vi "U3 eGetS Example.vi"() -> (0 "error out":errorcluster)   [LabVIEW 2020]
panel:
  in  "IOType":string="LJ_ioGET_AIN"
  in  "x1":i32=32
  in  "FirstFound":bool=TRUE
  in  "Address":string="1"
  in  "Value Write":dbl format="%.3f"
  out "Error Message":string="No Error"
  out "Value Read":dbl format="%.6f"
  in  "Channel #":i32
  # "IOTypes:\n\nLJ_ioGET_AIN = 10\nLJ_ioGET_AIN_DIFF = 15\nLJ_ioGET_AIN_ADVANCED = 16\nLJ_ioPUT_AIN_RANGE = 2000\nLJ_ioGET_AIN_RANGE = 2001\nLJ_ioPUT_ANALOG_ENABLE_BIT = 2013\nLJ_ioGET_ANALOG_ENABLE_BIT = 2014\nLJ_ioPUT_ANALOG_ENABLE_PORT = 2015\nLJ_ioGET_ANALOG_ENABLE_PORT = 2016\nLJ_ioPUT_DAC = 20\nLJ_ioPUT_DAC_ENABLE = 2002\nLJ_ioGET_DAC_ENABLE = 2003\nLJ_ioGET_DIGITAL_BIT = 30\nLJ_ioGET_DIGITAL_BIT_DIR = 31\nLJ_ioGET_DIGITAL_BIT_STATE = 32\nLJ_ioGET_DIGITAL_PORT = 35\nLJ_ioGET_DIGITAL_PORT_DIR = 36\nLJ_ioGET_DIGITAL_PORT_STATE = 37\nLJ_ioPUT_DIGITAL_BIT = 40\nLJ_ioPUT_DIGITAL_PORT = 45\nLJ_ioPUT_WAIT = 70\nLJ_ioGET_COUNTER = 50\nLJ_ioPUT_COUNTER_ENABLE = 2008\nLJ_ioGET_COUNTER_ENABLE = 2009\nLJ_ioPUT_COUNTER_RESET = 2012\nLJ_ioGET_TIMER = 60\nLJ_ioPUT_TIMER_VALUE = 2006\nLJ_ioPUT_TIMER_MODE = 2004\nLJ_ioGET_TIMER_MODE = 2005\nLJ_ioSHT_GET_READING = 500\nLJ_ioSPI_COMMUNICATION = 503\nLJ_ioI2C_COMMUNICATION = 504\nLJ_ioASYNCH_COMMUNICATION = 505\nLJ_ioTDAC_COMMUNICATION = 506\nLJ_ioPIN_CONFIGURATION_RESET = 2017\nLJ_ioRAW_OUT = 100\nLJ_ioRAW_IN = 101\nLJ_ioRAWMB_OUT = 104\nLJ_ioRAWMB_IN = 105\nLJ_ioSET_DEFAULTS = 103\nLJ_ioADD_STREAM_CHANNEL = 200\nLJ_ioADD_STREAM_CHANNEL_DIFF = 206\nLJ_ioCLEAR_STREAM_CHANNELS = 201\nLJ_ioSTART_STREAM = 202\nLJ_ioSTOP_STREAM = 203\nLJ_ioADD_STREAM_DAC = 207\nLJ_ioGET_STREAM_DATA = 204\nLJ_ioSET_STREAM_CALLBACK = 205\nLJ_ioSET_STREAM_CALLBACK_PTR = 260\nLJ_ioBUZZER = 300\nLJ_ioSET_EVENT_CALLBACK = 400\nLJ_ioPUT_CONFIG = 1000\nLJ_ioGET_CONFIG = 1001"
  # "Reads 1 input or writes 1 output.  Use \"U3 Pin Configuration Example.vi\" to set pins to digital\nor analog."
  # "Used for digital port IOtypes where\nx1 specifies the # of bits and then\nChannel # specifies starting channel.\nFor differential AIN, x1 specifies\nnegative channel."
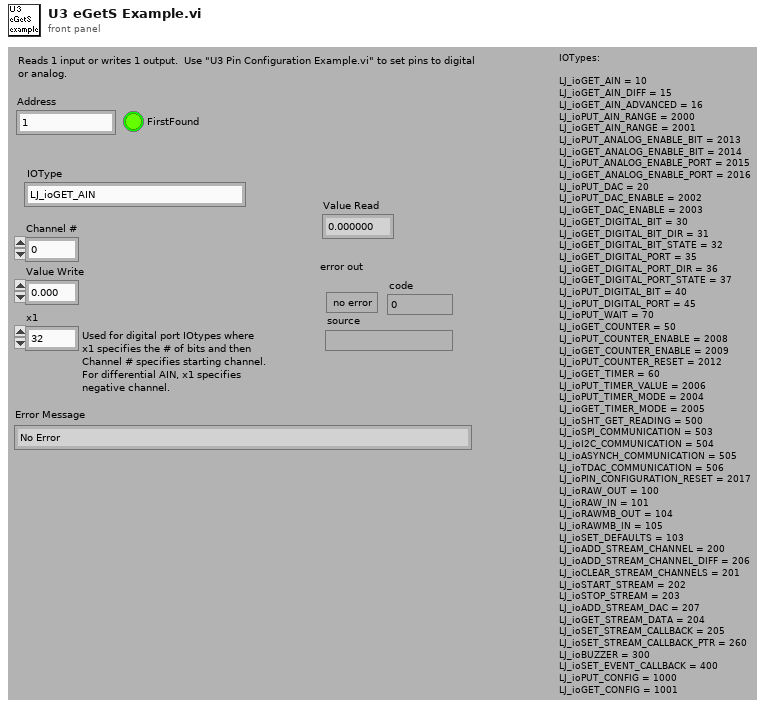
[diagram p1: front panel]
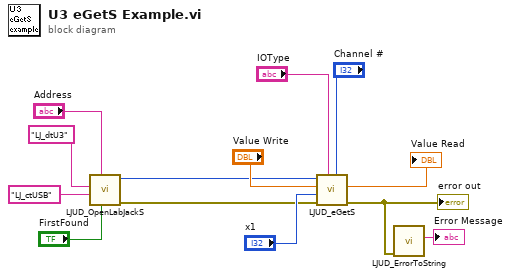
[diagram p0: block diagram]
diagram:
  n1 = call "LJUD_OpenLabJackS.vi"("FirstFound"="FirstFound", "Address"="Address", "ConnectionType"="LJ_ctUSB", "DeviceType"="LJ_dtU3") -> ("error out"=w2:errorcluster, "Handle"=w3:i32)  [unwired: 5 in, 1 out]
  n2 = call "LJUD_eGetS.vi"("Channel"="Channel #", "IOType"="IOType", "error in"=w2, "x1"="x1", "Value Write"="Value Write", "Handle In"=w3) -> ("error out"=w10:errorcluster, "Value Read"=→"Value Read":dbl)  [unwired: 3 in, 1 out]
  "error out" <- w10
  n3 = call "LJUD_ErrorToString.vi"("error in"=w10) -> ("String"=→"Error Message":string)  [unwired: 10 in]
